vi "write_data_rn.vi"(8 "error in (no error)":errorcluster, 10 "data":T1={"radius"=1.0, "mode"="connectivity", "return_distance"=TRUE, "sort_results"=FALSE}, 11 "RNeighbors in":refnum<class "RNeighbors.lvclass">) -> (0 "error out":errorcluster, 3 "RNeighbors out":refnum<class "RNeighbors.lvclass">)   [LabVIEW 2020, in "RNeighbors.lvclass"]
uses:
  RNeighbors.lvclass
  Controls/rneighbors_data.ctl
  RNeighbors.lvclass/RNeighbors.ctl
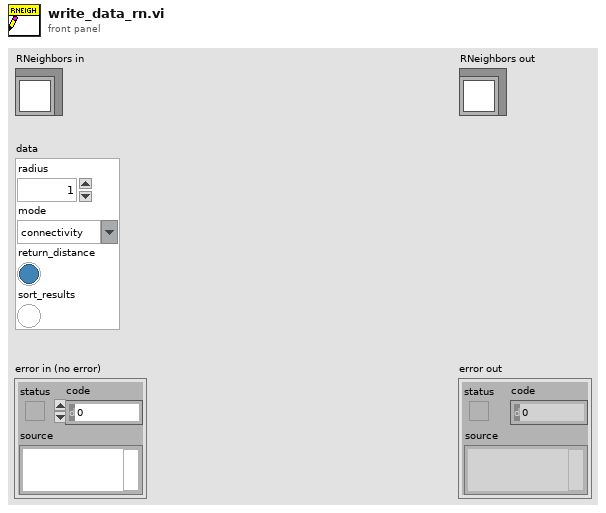
[diagram p1: front panel]
types:
  T1 = typedef "rneighbors_data.ctl" = cluster{"radius":dbl, "mode":string, "return_distance":bool, "sort_results":bool}
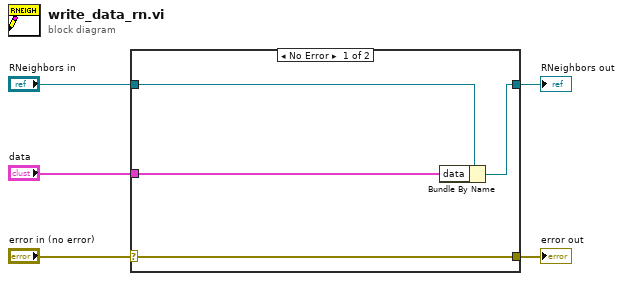
[diagram p0: block diagram]
diagram:
  n1 = case shown="No Error" "error in (no error)" {
    selector: "error in (no error)" -> [w9 w10]
    tunnel: [w9 w10] -> w4
    tunnel: [w7 w11] -> w2
    tunnel: "RNeighbors in" -> [w8 w11]
    tunnel: "data" -> [w6 _]
    frame No Error {
      n2 = Bundle By Name(cluster=w8, "data"=w6) -> (w7:refnum<class "RNeighbors.lvclass">)
    }
    frame Error {
    }
  }
  "error out" <- w4
  "RNeighbors out" <- w2
